vi "PWM Waveform PD500 Test.vi"(0 "Analysis Leg":i32, 1 "Board Selector":T2, 5 "Active Leg":i32, 9 "Waveform":waveform(dbl)[](array[waveform])) -> (4 "Inactive Values":T1, 6 "Active Values":T1)   [LabVIEW 2022 SP3]
uses:
  Serial Board Com/Board Select.ctl
  <vilib>/Analysis/Matrix/Datatypes/RealMatrix.ctl
  <vilib>/measure/mascope.llb/Pulse Measurements 1 chan.vi
  <vilib>/measure/madcrms.llb/Basic Averaged DC-RMS for 1 Chan.vi
  <vilib>/measure/NI_MAPro.lvlib
  <vilib>/Analysis/Matrix/NI_Matrix.lvlib
panel:
  out "error out":errorcluster
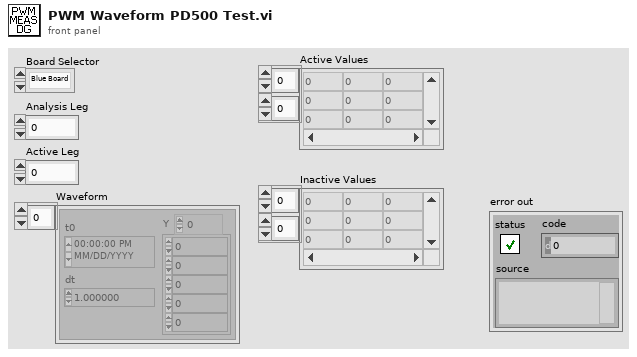
[diagram p1: front panel]
types:
  T1 = typedef "NI_Matrix.lvlib/RealMatrix.ctl" = dbl[][]
  T2 = typedef "Board Select.ctl" = enum16{"Blue Board", "Green Board"}
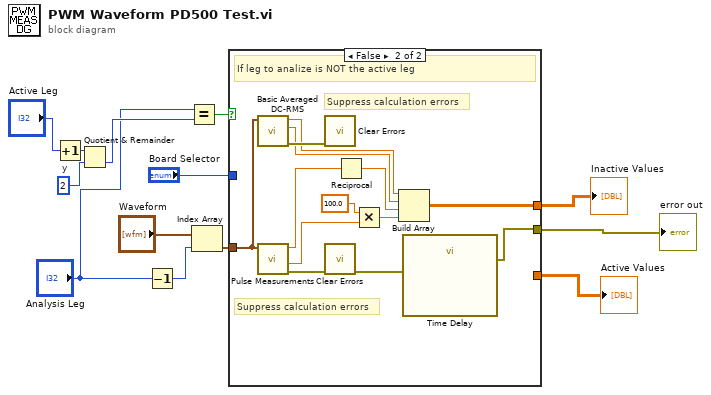
[diagram p0: block diagram]
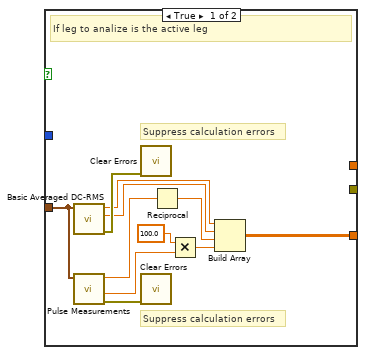
[diagram p2: hidden frame]
diagram:
  w7 = 2  # y
  n1 = Increment(x="Active Leg") -> (x+1=w6:i32)
  n2 = Quotient & Remainder(x=w6, y=w7) -> (floor(x/y)=w4:i32)  [unwired: 1 out]
  n3 = Decrement(x="Analysis Leg") -> (x-1=w1:i32)
  n4 = Equal?(x="Analysis Leg", y=w4) -> (x = y?=w11:bool)
  n5 = Index Array(array="Waveform", index=w1) -> (element=w12:waveform(dbl))
  n6 = case shown="False" w11 {
    tunnel: w12 -> [w19 w32]
    tunnel: "Board Selector" -> [_ _]
    tunnel: [_ w27] -> w9
    tunnel: [w14 _] -> w8
    tunnel: [_ w25] -> w3
    frame True {
      # "Suppress calculation errors"
      # "Suppress calculation errors"
      # "If leg to analize is the active leg"
      n7 = call-poly <vilib>:"Basic Averaged DC-RMS.vi"("signal in"=w19) -> ("error out"=w20:errorcluster, "RMS value"=w17:dbl, "DC value"=w18:dbl)  [unwired: 7 in, 1 out]
      n8 = call-poly <vilib>:"Pulse Measurements.vi"("signal in"=w19) -> ("error out"=w21:errorcluster, "duty cycle"=w23:dbl, "period"=w22:dbl)  [unwired: 6 in, 2 out]
      n9 = call <vilib>:"Clear Errors.vi"("error in (no error)"=w20) -> ()  [unwired: 5 in, 2 out]
      n10 = call <vilib>:"Clear Errors.vi"("error in (no error)"=w21) -> ()  [unwired: 5 in, 2 out]
      n11 = Reciprocal(x=w22) -> (1/x=w16:dbl)
      n12 = Multiply(x=100.0, y=w23) -> (x*y=w15:dbl)
      n13 = Build Array(w18, w17, w16, w15) -> (w14:T1)
    }
    frame False {
      # "Suppress calculation errors"
      # "Suppress calculation errors"
      # "If leg to analize is NOT the active leg"
      n14 = call-poly <vilib>:"Basic Averaged DC-RMS.vi"("signal in"=w32) -> ("error out"=w33:errorcluster, "RMS value"=w30:dbl, "DC value"=w31:dbl)  [unwired: 7 in, 1 out]
      n15 = call-poly <vilib>:"Pulse Measurements.vi"("signal in"=w32) -> ("error out"=w34:errorcluster, "duty cycle"=w36:dbl, "period"=w35:dbl)  [unwired: 6 in, 2 out]
      n16 = call <vilib>:"Clear Errors.vi"("error in (no error)"=w33) -> ()  [unwired: 5 in, 2 out]
      n17 = call <vilib>:"Clear Errors.vi"("error in (no error)"=w34) -> ("error out"=w26:errorcluster)  [unwired: 5 in, 1 out]
      n18 = Reciprocal(x=w35) -> (1/x=w29:dbl)
      n19 = Multiply(x=100.0, y=w36) -> (x*y=w28:dbl)
      n20 = Build Array(w31, w30, w29, w28) -> (w27:T1)
      n21 = call "Time Delay"("error in (no error)"=w26) -> ("error out"=w25:errorcluster)  [unwired: 10 in]
    }
  }
  "Inactive Values" <- w9
  "Active Values" <- w8
  "error out" <- w3
